vi "Resample Waveform (continuous).vi"(0 "waveform in":waveform(dbl), 1 "reset":bool, 5 "dt":dbl=1.0 format="%.2p", 7 "t0":timestamp=timestamp(-9223372036854775808 s since 1904-01-01) format="%<%.4X>T", 9 "interpolation mode":u16(ring)=1 items=["coerce", "linear", "spline", "FIR filter"], 11 "error in (no error)":errorcluster, 12 "FIR filter specifications":T1={"alias rejection (dB)"=120.0, "normalized bandwidth"=0.4536} {"normalized bandwidth" format="%.4f"; "alias rejection (dB)" format="%.2f"}) -> (4 "resampled waveform out":waveform(dbl), 8 "next t0":timestamp=timestamp(-9223372036854775808 s since 1904-01-01) format="%<%.4X>T", 10 "used t0":timestamp=timestamp(-9223372036854775808 s since 1904-01-01) format="%<%.4X>T", 14 "t0 adjusted warning":bool, 15 "error out":errorcluster)   [LabVIEW 2020, in "NI_MAPro.lvlib"]
doc: "Resamples an input waveform according to the user-defined values for <B>t0</B> and <B>dt</B>. Wire data to the <B>waveform in</B> input to determine the polymorphic instance to use or manually select the instance."
uses:
  NI_MAPro.lvlib
  NI_MABase.lvlib
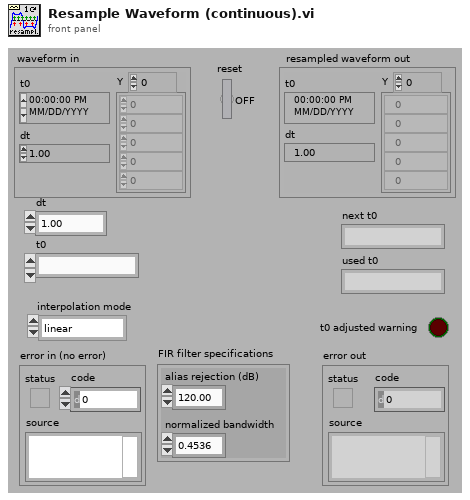
[diagram p1: front panel]
types:
  T1 = cluster{"alias rejection (dB)":dbl, "normalized bandwidth":dbl}
  T2 = cluster{"scaled filter":dbl[], "sub-filter size":i32, "filter max index":i32, "FIR index step":dbl, "half duration":dbl}
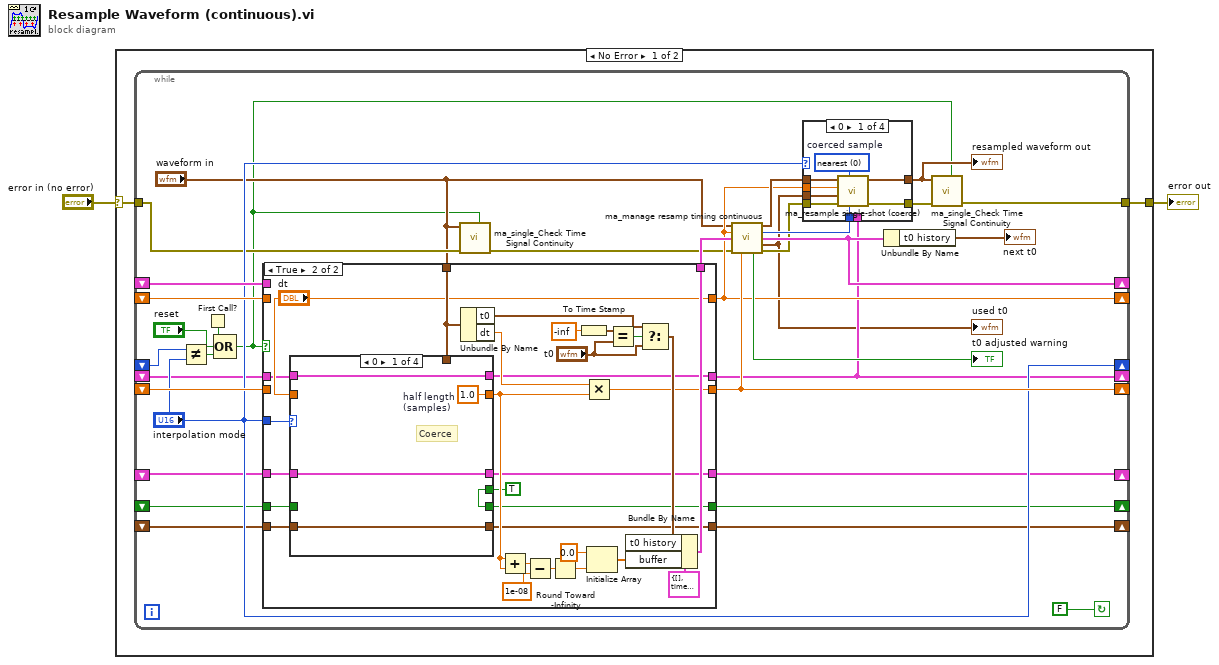
[diagram p0: block diagram]
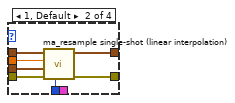
[diagram p2: hidden frame]
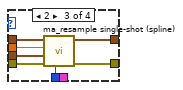
[diagram p3: hidden frame]
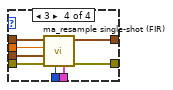
[diagram p4: hidden frame]
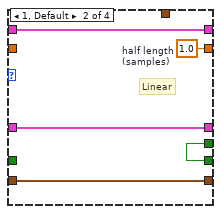
[diagram p6: hidden frame]
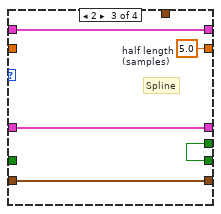
[diagram p7: hidden frame]
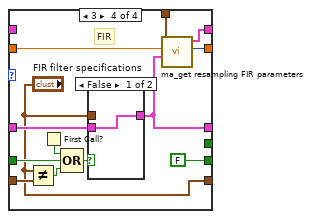
[diagram p8: hidden frame]
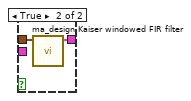
[diagram p9: hidden frame]
diagram:
  n1 = case shown="No Error" "error in (no error)" {
    selector: "error in (no error)" -> [w3 w136]
    tunnel: [w4 w136] -> w2
    frame No Error {
      n2 = while {
        shift-right: [w31] -> _
        shift-left: _ -> [w34]
        shift-right: ["interpolation mode"] -> _
        shift-left: _ -> [w37]
        shift-right: [w33] -> _
        shift-left: _ -> [w32]
        shift-right: [w22] -> _
        shift-left: _ -> [w29]
        shift-right: [w21] -> _
        shift-left: _ -> [w20]
        tunnel: [w9] -> w4
        tunnel: w3 -> [w13]
        shift-right: [w19] -> _
        shift-left: _ -> [w18]
        shift-right: [w16] -> _
        shift-left: _ -> [w17]
        shift-right: [w14] -> _
        shift-left: _ -> [w15]
        stop <- FALSE continue-if-true
        n3 = Not Equal?(x=w37, y="interpolation mode") -> (x != y?=w36:bool)
        n4 = First Call?() -> (First Call?: T/F=w24:bool)
        n5 = Compound Arithmetic op=OR(w24, "reset", w36) -> (w5:bool)
        n6 = case shown="True" w5 {
          tunnel: [w74 w99] -> w33
          tunnel: "interpolation mode" -> [_ w87]
          tunnel: [w75 w101] -> w35
          tunnel: w34 -> [w75 _]
          tunnel: w32 -> [w74 _]
          tunnel: [w73 "dt"] -> w22
          tunnel: w29 -> [w73 _]
          tunnel: [w72 w93] -> w21
          tunnel: w20 -> [w72 w90]
          tunnel: "waveform in" -> [_ w92]
          tunnel: [w71 w89] -> w19
          tunnel: w18 -> [w71 w88]
          tunnel: w17 -> [w70 w85]
          tunnel: [w70 w84] -> w16
          tunnel: w15 -> [w69 w83]
          tunnel: [w69 w82] -> w14
          frame False {
          }
          frame True {
            n7 = case shown="0" w87 {
              tunnel: [w109 w114 w119 w132] -> w94
              tunnel: [w108 w113 w115 w131] -> w93
              tunnel: w90 -> [w108 w113 w115 _]
              tunnel: w92 -> [_ _ _ w130]
              tunnel: "dt" -> [_ _ _ w129]
              tunnel: [w107 w112 w118 w128] -> w89
              tunnel: w88 -> [w107 w112 w118 w127]
              tunnel: [w106 w111 w117 FALSE] -> w84
              tunnel: w85 -> [_ _ _ w123]
              tunnel: TRUE -> [w106 w111 w117 _]
              tunnel: [w105 w110 w116 "FIR filter specifications"] -> w82
              tunnel: w83 -> [w105 w110 w116 w125]
              frame 0 {
                w109 = 1.0  # half length (samples)
                # "Coerce"
              }
              frame 1, Default {
                w114 = 1.0  # half length (samples)
                # "Linear"
              }
              frame 2 {
                w119 = 5.0  # half length (samples)
                # "Spline"
              }
              frame 3 {
                # "FIR"
                n8 = Not Equal?(x="FIR filter specifications", y=w125) -> (x != y?=w124:bool)
                n9 = First Call?() -> (First Call?: T/F=w121:bool)
                n10 = Compound Arithmetic op=OR(w121, w123, w124) -> (w126:bool)
                n11 = case shown="False" w126 {
                  tunnel: [w133 w135] -> w128
                  tunnel: "FIR filter specifications" -> [_ w134]
                  tunnel: w127 -> [w133 _]
                  frame False {
                  }
                  frame True {
                    n12 = call "ma_design Kaiser windowed FIR filter.vi"("FIR filter specifications"=w134) -> ("filter data"=w135:cluster{"h":dbl[], "Max Decimation":dbl})  [unwired: 8 in, 1 out]
                  }
                }
                n13 = call "ma_get resampling FIR parameters.vi"("filter info"=w128, "dt"=w129, "Waveform in"=w130) -> ("history size"=w132:i32, "Filter parameters"=w131:T2)  [unwired: 7 in]
              }
            }
            n14 = Unbundle By Name(w92) -> ("t0"=w79:timestamp, "dt"=w104:dbl)
            n15 = Add(x=w94, y=w94) -> (x+y=w98:dbl)
            n16 = Subtract(x=w98, y=1e-08) -> (x-y=w96:dbl)
            n17 = Round Toward -Infinity(1:w96) -> (0:w95:dbl)
            n18 = To Time Stamp(1:-inf ("x")) -> (0:w77:timestamp)
            n19 = Multiply(x=w104, y=w94) -> (x*y=w99:dbl)
            n20 = Initialize Array(0.0 ("element"), w95) -> (w102:dbl[])
            n21 = Equal?(x=w77, y="t0") -> (x = y?=w81:bool)
            n22 = Select(t=w79, s=w81, f="t0") -> (s? t:f=w100:timestamp)
            n23 = Bundle By Name(cluster=cluster{"buffer":dbl[], "t0 history":timestamp} {"buffer"=[], "t0 history"=timestamp(0 s since 1904-01-01)} ("state info out"), "t0 history"=w100, "buffer"=w102) -> (w101:cluster{"buffer":dbl[], "t0 history":timestamp})
          }
        }
        n24 = call "ma_single_Check Time Signal Continuity.vi"("Ignore input time stamp"=w5, "error in (no error)"=w13, "Waveform"="waveform in") -> ("error out"=w6:errorcluster)  [unwired: 5 in, 3 out]
        n25 = call "ma_manage resamp timing continuous.vi"("waveform in"="waveform in", "dt"=w22, "state info in"=w35, "error in"=w6, "filter half-length (s)"=w33) -> ("waveform to be processed"=w27:waveform(dbl), "#elements"=w26:i32, "state info out"=w31:cluster{"buffer":dbl[], "t0 history":timestamp}, "used t0"=w8:timestamp, "t0 adjusted warning"=→"t0 adjusted warning":bool, "error out"=w23:errorcluster)  [unwired: 5 in]
        "used t0" <- w8
        n26 = case shown="0" "interpolation mode" {
          tunnel: w27 -> [w46 w53 w60 w68]
          tunnel: w26 -> [w39 w47 w54 w62]
          tunnel: w8 -> [w45 w52 w59 w67]
          tunnel: w22 -> [w44 w51 w58 w66]
          tunnel: w23 -> [w43 w50 w57 w65]
          tunnel: [w42 w49 w56 w64] -> w10
          tunnel: [w41 w48 w55 w63] -> w11
          tunnel: w21 -> [_ _ _ w61]
          frame 0 {
            w40 = u16 0 items=["nearest", "previous", "next"]  # coerced sample
            n27 = call "ma_resample single-shot (coerce).vi"("#elements"=w39, "coerced sample"=w40, "error in"=w43, "t0"=w45, "dt"=w44, "waveform in"=w46) -> ("error out"=w42:errorcluster, "resampled waveform out"=w41:waveform(dbl))  [unwired: 4 in]
          }
          frame 1, Default {
            n28 = call "ma_resample single-shot (linear interpolation).vi"("#elements"=w47, "error in"=w50, "t0"=w52, "dt"=w51, "waveform in"=w53) -> ("error out"=w49:errorcluster, "resampled waveform out"=w48:waveform(dbl))  [unwired: 5 in]
          }
          frame 2 {
            n29 = call "ma_resample single-shot (spline).vi"("#elements"=w54, "error in"=w57, "t0"=w59, "dt"=w58, "waveform in"=w60) -> ("error out"=w56:errorcluster, "resampled waveform out"=w55:waveform(dbl))  [unwired: 3 in, 2 out]
          }
          frame 3 {
            n30 = call "ma_resample single-shot (FIR).vi"("Filter parameters"=w61, "#elements"=w62, "error in"=w65, "t0"=w67, "dt"=w66, "waveform in"=w68) -> ("error out"=w64:errorcluster, "resampled waveform out"=w63:waveform(dbl))  [unwired: 4 in]
          }
        }
        "resampled waveform out" <- w11
        n31 = Unbundle By Name(w31) -> ("t0 history"=→"next t0":timestamp)
        n32 = call "ma_single_Check Time Signal Continuity.vi"("Ignore input time stamp"=w5, "error in (no error)"=w10, "Waveform"=w11) -> ("error out"=w9:errorcluster)  [unwired: 5 in, 3 out]
      }
    }
    frame Error {
    }
  }
  "error out" <- w2
